vi "get segment values from XY data.vi"() -> ()   [LabVIEW 2013]
panel:
  in  "appended array 2":dbl[][](array[numeric])
  in  "speed":u32(slide)
  out "Image 3":T1(plugin-control)
  in  "AVI Path":path=path "E:/PhD work/PhD research work/Videos/Chen Jin vs Hu Yun (Edited).avi"
  in  "appended array":dbl[][](array[numeric])=array1939x5[9695 elements]
  in  "Frames XY (top/bottom)":dbl[][](array[numeric])
  out "Infered action indicators":string[][](array[string])
  out "Movement data from both players":i32[][](array[numeric])
  out "Top player court segment display 2":bool[][](array[boolean])
  out "count top":i32[](graph)
  out "count bottom":i32[](graph)
  out "trans top":i32[](graph)
  out "trans bottom":i32[](graph)
  in  "ON":bool
  out "Top player court segment display":bool[][](array[boolean])
  out "Top VIew":cluster{"Numeric":dbl, "Numeric":dbl}[](graph)
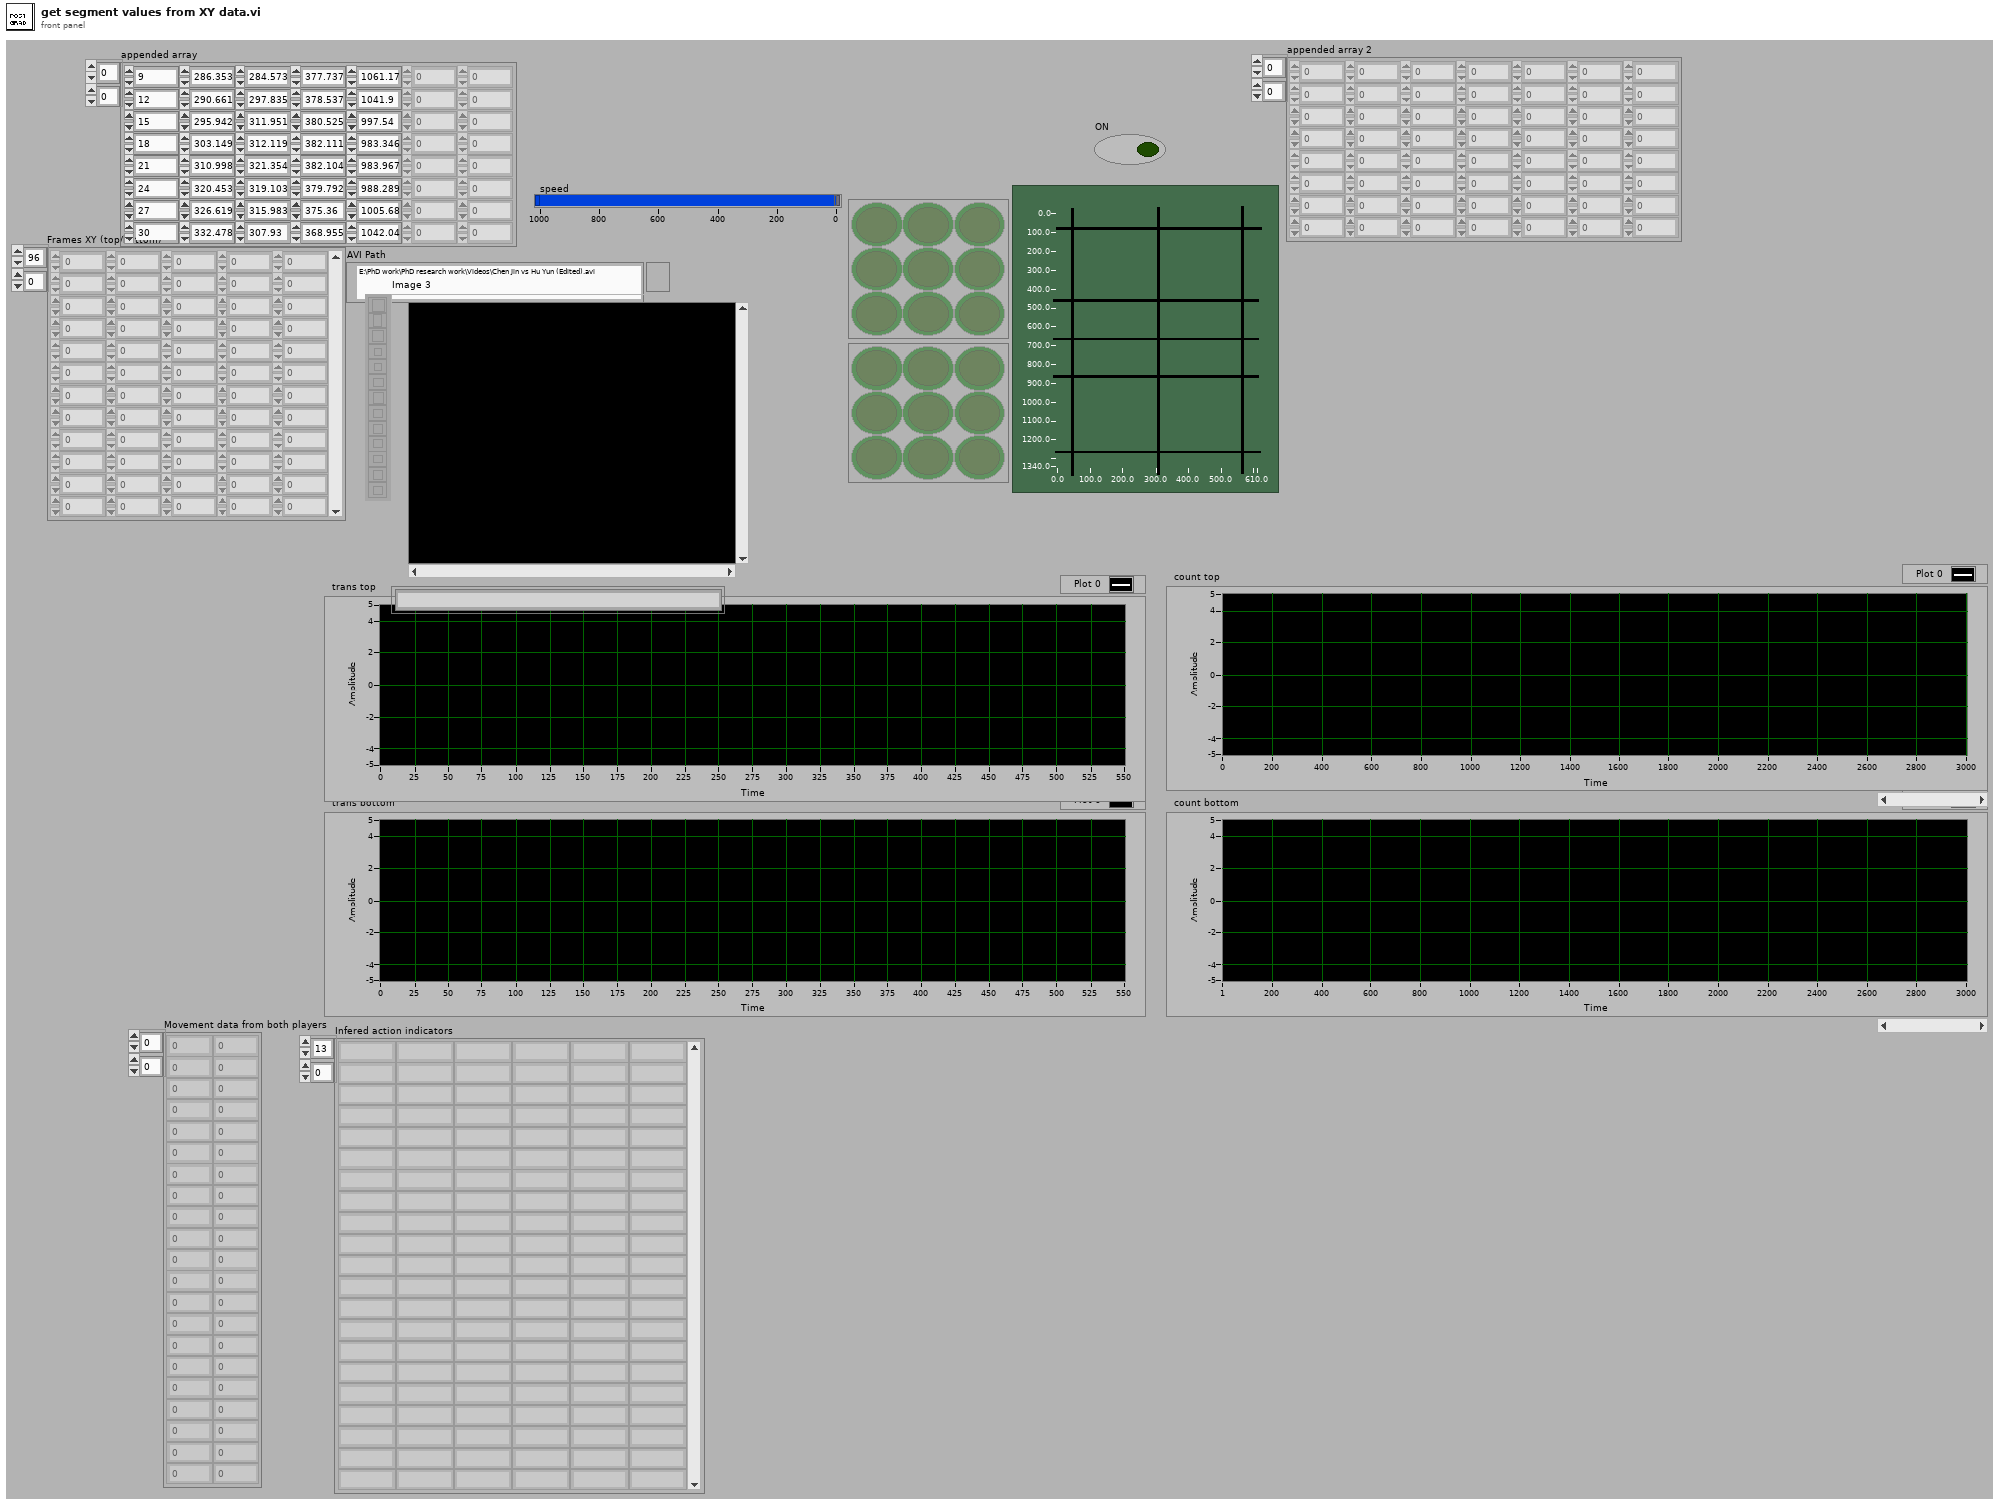
[diagram p1: front panel]
types:
  T1 = typedef "IMAQ Image.ctl" = refnum<image>
  T2 = typedef "Image Type" = u32
  T3 = typedef "AviRefnum.ctl" = refnum<k1>
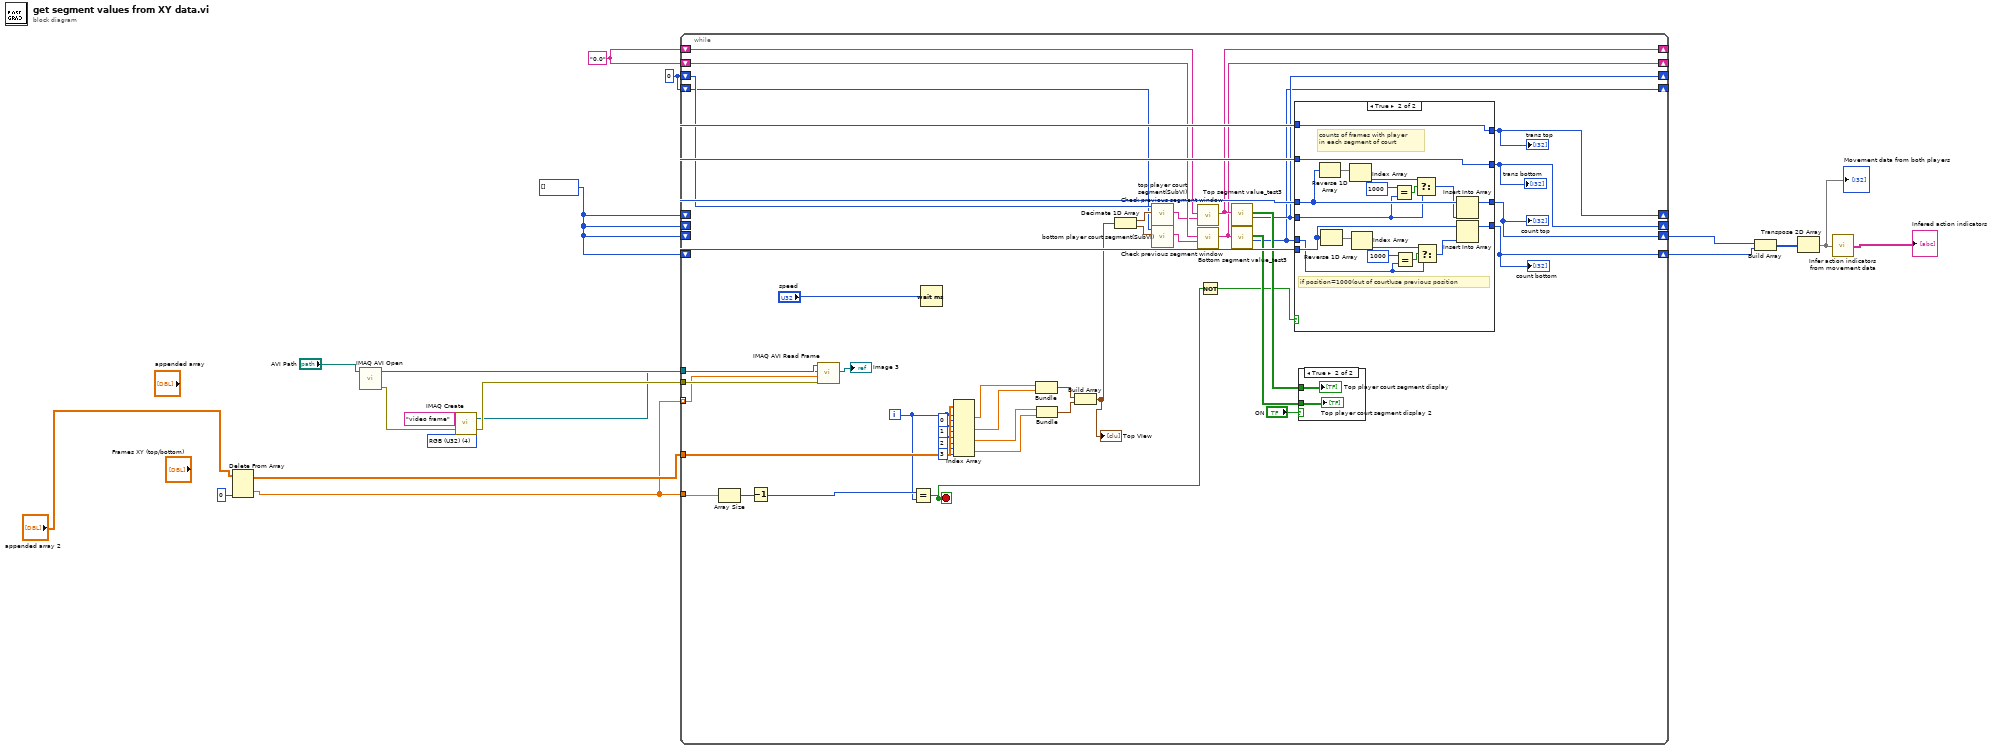
[diagram p0: block diagram]
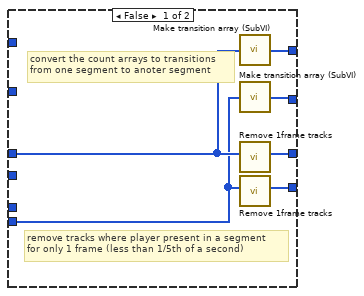
[diagram p2: hidden frame]
diagram:
  w2 = 0 ("Top player segment value")
  w8 = T2 4 items=["Grayscale (U8)", "Grayscale (I16)", "Grayscale (SGL)", "Complex (CSG)", "RGB (U32)", "HSL (U32)", "RGB (U64)", "Grayscale (U16)"] ("Image Type")
  w19 = "0,0" ("Player segment position")
  w18 = i32[] [] ("input array")
  n1 = Delete From Array(array="appended array 2", index (col)=0 ("disabled index (col)")) -> (deleted portion=w3:dbl[], array with subset deleted=w11:dbl[][])  [unwired: 2 in]
  n2 = call "IMAQ AVI Open"("AVI Path"="AVI Path") -> ("error out"=w6:errorcluster, "Avi Refnum"=w9:T3)  [unwired: 9 in]
  n3 = call "IMAQ Create"("Image Name"="video frame", "Image Type"=w8, "error in (no error)"=w6) -> ("New Image"=w4:T1, "error out"=w5:errorcluster)  [unwired: 2 in]
  n4 = while {
    shift-right: [w46] -> w14
    shift-left: w18 -> [w61]
    shift-right: [w47] -> w13
    shift-left: w18 -> [w62]
    shift-right: [w53] -> _
    shift-left: w18 -> [w59]
    shift-right: [w58] -> _
    shift-left: w18 -> [w60]
    shift-right: [w49] -> _
    shift-left: w19 -> [w54]
    shift-right: [w50] -> _
    shift-left: w19 -> [w55]
    tunnel: w3 -> [w36]
    tunnel: w11 -> [w45]
    tunnel: w9 -> [w29]
    tunnel: w5 -> [w28]
    tunnel: w4 -> [w27]
    tunnel: w3 -> [w26] mode=indexing
    shift-right: [w23] -> _
    shift-left: w2 -> [w21]
    shift-right: [w22] -> _
    shift-left: w2 -> [w20]
    i -> [w33]
    stop <- w31 stop-if-true
    n5 = Array Size(array=w36) -> (size(s)=w35:i32)
    n6 = Decrement(x=w35) -> (x-1=w34:i32)
    n7 = call "IMAQ AVI Read Frame"("error in (no error)"=w28, "Frame Number"=w26, "Image"=w27, "Avi Refnum"=w29) -> ("Image Out"=→"Image 3":T1)  [unwired: 4 in, 3 out]
    n8 = Equal?(x=w34, y=w33) -> (x = y?=w31:bool)
    n9 = Wait (ms)(milliseconds to wait="speed") -> ()  [unwired: 1 out]
    n10 = Index Array(array=w45, index (row) #1=w33, index (col) #1=0 ("disabled index (col)"), index (row) #2=w33, index (col) #2=1 ("disabled index (col)"), index (row) #3=w33, index (col) #3=2 ("disabled index (col)"), index (row) #4=w33, index (col) #4=3 ("disabled index (col)")) -> (element #1=w40:dbl, element #2=w39:dbl, element #3=w38:dbl, element #4=w37:dbl)
    n11 = Bundle("Numeric"=w40, "Numeric"=w39) -> (w66:cluster{"Numeric":dbl, "Numeric":dbl})  [unwired: 1 in]
    n12 = Bundle("Numeric"=w38, "Numeric"=w37) -> (w48:cluster{"Numeric":dbl, "Numeric":dbl})  [unwired: 1 in]
    n13 = Build Array(w66, w48) -> (w30:cluster{"Numeric":dbl, "Numeric":dbl}[])
    "Top VIew" <- w30
    n14 = Decimate 1D Array(w30) -> (w64:cluster{"Numeric":dbl, "Numeric":dbl}[], w65:cluster{"Numeric":dbl, "Numeric":dbl}[])
    n15 = call "top player court segment(SubVI).vi"("Top player position"=w64, "previous segment"=w21) -> ("Top player segment position"=w52:string)  [unwired: 9 in]
    n16 = call "bottom player court segment(SubVI).vi"("Bottom player position"=w65, "previous segment"=w20) -> ("Bottom player segment position"=w51:string)  [unwired: 9 in]
    n17 = call "Check previous segment window.vi"("Current player segment position"=w52, "Previous player segment position"=w55) -> ("Player segment position"=w50:string)  [unwired: 9 in]
    n18 = call "Check previous segment window.vi"("Current player segment position"=w51, "Previous player segment position"=w54) -> ("Player segment position"=w49:string)  [unwired: 9 in]
    n19 = Not(x=w31) -> (.not. x?=w32:bool)
    n20 = call "Top segment value_test3.vi"("Top player segment position"=w50) -> ("Top player segment value"=w23:i32, "Top player court segment display"=w57:bool[][])  [unwired: 9 in]
    n21 = call "Bottom segment value_test3.vi"("Bottom player segment position"=w49) -> ("Bottom player segment"=w22:i32, "Bottom player court segment display"=w56:bool[][])  [unwired: 9 in]
    n22 = case shown="True" w32 {
      tunnel: w62 -> [w70 w86]
      tunnel: w61 -> [w69 w76]
      tunnel: [w71 w87] -> w53
      tunnel: [w72 w88] -> w58
      tunnel: w22 -> [_ w73]
      tunnel: w23 -> [_ w81]
      tunnel: w60 -> [_ w88]
      tunnel: w59 -> [_ w87]
      tunnel: [w68 w90] -> w46
      tunnel: [w67 w89] -> w47
      frame False {
        # "convert the count arrays to transitions \nfrom one segment to anoter segment"
        # "remove tracks where player present in a segment \nfor only 1 frame (less than 1/5th of a second)"
        n23 = call "Make transition array (SubVI).vi"("count array in"=w70) -> ("Transition array out"=w71:i32[])
        n24 = call "Make transition array (SubVI).vi"("count array in"=w69) -> ("Transition array out"=w72:i32[])
        n25 = call "Remove 1frame tracks.vi"("count array in"=w70) -> ("count array out"=w67:i32[])  [unwired: 10 in]
        n26 = call "Remove 1frame tracks.vi"("count array in"=w69) -> ("count array out"=w68:i32[])  [unwired: 10 in]
      }
      frame True {
        # "if position=1000(out of court)use previous position"
        # "counts of frames with player\nin each segment of court"
        n27 = Reverse 1D Array(array=w86) -> (reversed array=w85:i32[])
        n28 = Reverse 1D Array(array=w76) -> (reversed array=w75:i32[])
        n29 = Index Array(array=w85) -> (element=w82:i32)  [unwired: 1 in]
        n30 = Index Array(array=w75) -> (element=w79:i32)  [unwired: 1 in]
        n31 = Equal?(x=1000 ("y"), y=w81) -> (x = y?=w83:bool)
        n32 = Equal?(x=1000 ("y"), y=w73) -> (x = y?=w78:bool)
        n33 = Select(t=w82, s=w83, f=w81) -> (s? t:f=w80:i32)
        n34 = Select(t=w79, s=w78, f=w73) -> (s? t:f=w74:i32)
        n35 = Insert Into Array(array=w86, new element=w80) -> (w89:i32[])  [unwired: 1 in]
        n36 = Insert Into Array(array=w76, new element=w74) -> (w90:i32[])  [unwired: 1 in]
      }
    }
    "trans bottom" <- w58
    "trans top" <- w53
    "count bottom" <- w46
    "count top" <- w47
    n37 = case shown="True" "ON" {
      tunnel: w57 -> [_ w92]
      tunnel: w56 -> [_ w91]
      frame False {
      }
      frame True {
        "Top player court segment display" <- w92
        "Top player court segment display 2" <- w91
      }
    }
  }
  n38 = Build Array(w13, w14) -> (w17:i32[][])
  n39 = Transpose 2D Array(2D array=w17) -> (transposed array=w15:i32[][])
  "Movement data from both players" <- w15
  n40 = call "Infer action indicators from movement data.vi"("movement data from both players"=w15) -> ("Infered action indicators"=→"Infered action indicators":string[][])
